vi "TIO RPC Blocking.vi"(8 "error in (no error)":errorcluster, 9 "Payload":string, 10 "Named Method":string="mcu.desc", 11 "TS Connection":T1={"Type"=enum."TCP", "URL"="serial:///dev/cu.usbserial-00000", "TCP"=refnum, "Timeout"=500, "Route"="", "UDP"=refnum}) -> (0 "error out":errorcluster={"status"=TRUE, "code"=-1073807252, "source"="VISA Read in SLIP Decode Serial Read.vi->NN VISA Read.vi->NN RPC.vi"}, 1 "Response":bool, 2 "Respose":string, 3 "TS Connection":T1={"Type"=enum."TCP", "URL"="serial:///dev/cu.usbserial-00000", "TCP"=refnum, "Timeout"=500, "Route"="", "UDP"=refnum})   [LabVIEW 2017]
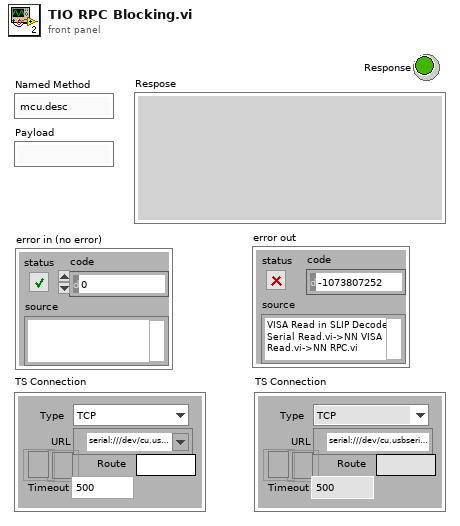
[diagram p1: front panel]
types:
  T1 = cluster{"Type":enum16{"TCP", "UDP", "Serial"}, "URL":refnum<visa-resource-name>, "TCP":refnum<k5>, "Timeout":u32, "Route":string, "UDP":refnum<k16>}
  T2 = enum8{"Invalid", "Log", "RPC Request", "RPC Reply", "RPC Error", "Stream Description", "User"}
  T3 = cluster{"Type":enum16{"TCP", "Serial"}, "URL":refnum<visa-resource-name>, "TCP":refnum<k5>, "Timeout":u32, "Route":string}
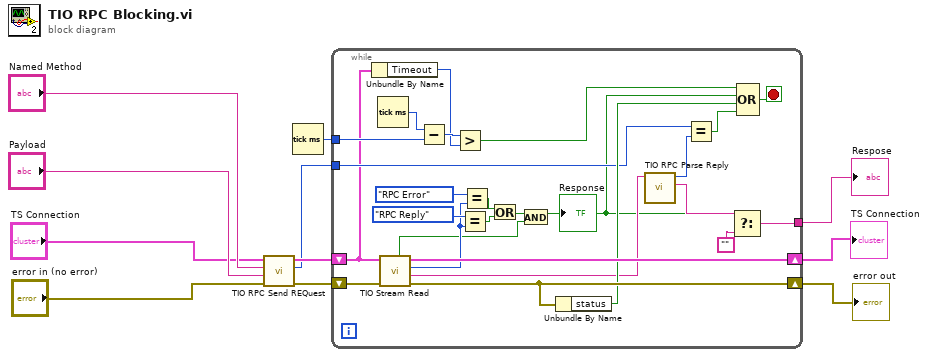
[diagram p0: block diagram]
diagram:
  n1 = call <instrlib>:"TIO RPC Send REQuest.vi"("error in (no error)"="error in (no error)", "Payload"="Payload", "Topic"="Named Method", "TS Connection"="TS Connection") -> ("error out"=w11:errorcluster, "Request ID"=w1:u16, "TS Connection"=w9:T1)  [unwired: 5 in]
  n2 = Tick Count (ms)() -> (millisecond timer value=w6:u32)
  n3 = while {
    shift-right: [w32] -> w10
    shift-left: w11 -> [w37]
    shift-right: [w36] -> w3
    shift-left: w9 -> [w15]
    tunnel: w6 -> [w34]
    tunnel: [w26] -> w2
    tunnel: w1 -> [w24]
    stop <- w29 stop-if-true
    n4 = Unbundle By Name(w15) -> ("Timeout"=w28:u32)
    n5 = Tick Count (ms)() -> (millisecond timer value=w35:u32)
    n6 = call <instrlib>:"TIO Stream Read.vi"("error in (no error)"=w37, "TS Connection"=w15) -> ("error out"=w32:errorcluster, "Payload"=w22:string, "Type"=w18:T2, "TS Connection"=w36:T3, "Routing Matches"=w12:bool)  [unwired: 4 in, 1 out]
    n7 = Subtract(x=w35, y=w34) -> (x-y=w33:u32)
    n8 = Greater?(x=w33, y=w28) -> (0:w31:bool)
    n9 = Equal?(x=T2."RPC Reply" ("Type"), y=w18) -> (x = y?=w16:bool)
    n10 = Equal?(x=T2."RPC Error" ("Type"), y=w18) -> (x = y?=w17:bool)
    n11 = Or(x=w17, y=w16) -> (x .or. y?=w14:bool)
    n12 = And(x=w14, y=w12) -> (x .and. y?=w13:bool)
    "Response" <- w13
    n13 = Unbundle By Name(w32) -> ("status"=w30:bool)
    n14 = call <instrlib>:"TIO RPC Parse Reply.vi"("Payload"=w22) -> ("Payload"=w20:string, "Request ID"=w21:u16)  [unwired: 9 in]
    n15 = Equal?(x=w24, y=w21) -> (x = y?=w23:bool)
    n16 = Select(t=w20, s=w13, f="") -> (s? t:f=w26:string)
    n17 = Compound Arithmetic op=OR(w31, w13, w30, w23) -> (w29:bool)
  }
  "error out" <- w10
  "Respose" <- w2
  "TS Connection" <- w3
